vi "220125_xiang_calibration data analysis.vi"() -> ()   [LabVIEW 2020]
uses:
  OldDAQtask/CylinderCalibration/XYZE_power_spectra.ctl
  OldDAQtask/CylinderCalibration/single_power_spectrum.ctl
  OldDAQtask/CylinderCalibration/XYZ scan data.ctl
  OldDAQtask/CylinderCalibration/fast winding result.ctl
  <vilib>/Analysis/baseanly.llb/Mean (DBL).vi
  <vilib>/Utility/file.llb/Write Delimited Spreadsheet (DBL).vi
  OldDAQtask/HeightFinder/HeightFinder.lvlib
  <vilib>/Analysis/NI_AALBase.lvlib
  OldDAQtask/CylinderCalibration/CylinderCalibration.lvlib
  <vilib>/Analysis/NI_AALPro.lvlib
panel:
  out "ellipticity fitting 4":cluster{dbl[], dbl[]}[](graph)
  out "ellipticity fitting 3":cluster{dbl[], dbl[]}[](graph)
  out "ellipticity fitting 2":cluster{dbl[], dbl[]}[](graph)
  out "ellipticity fitting":cluster{dbl[], dbl[]}[](graph)
  out "error out":errorcluster
  out "pb1":dbl(slide)=1.0 scale=0.0..1.0
  in  "kT_pNnm":dbl=4.09
  in  "stop":bool
  in  "cylinder list":i32[](listbox)
  in  "root path":path=path "Y:/Setup4/xg237/220124_xg237_calibration Q30"
  in  "Tab Control":T1(tab)
  out "result":T2
  out "Height finder data":cluster{dbl[], "Best Polynomial Fit":dbl[]}[](graph)
  out "original calibration file":string="[Trap and cylinder calibration]\nKz, pN/nm/W=0.349554\nKx, pN/nm/W=0.376339\nKy, pN/nm/W=0.248999\nSz, 1/nm=0.000578\nSx, 1/nm=0.000761\nSy, 1/nm=0.000667\nKang, pNnm/rad/W=17149.300335\nMax ellipticity, 1=0.032157\nFocal shift=0.790000\nZsignalHeightDependence, 1/nm=0\n[Piezo AO calibration and settings]\nVx/Px(V/nm)=0.000667\nVy/Py(V/nm)=0.000667\nVz/Pz(V/nm)=0.002000\nMax Px (nm)=30000.000000\nMax Py (nm)=30000.000000\nMax Pz (nm)=10000.000000\nMin Px (nm)=0.000000\nMin Py (nm)=0.000000\nMin Pz (nm)=0.000000\nVx0 (V)=-10.000000\nVy0 (V)=-10.000000\nVz0 (V)=-10.000000\nAI2p=1.101000E+4\\095.746000E+3\\093.323000E+0\\0D\\0A1.016000E+4\\095.766000E+3\\093.739000E+0\\0D\\0A6.154000E+3\\095.319000E+3\\091.621000E+1\\0D\\0A\n[matrix Mp2s (3X3)]\na11=1.000000\na12=0.000000\na13=0.000000\na21=0.000000\na22=1.000000\na23=0.000000\na31=0.000000\na32=0.000000\na33=1.000000\n[DAQ settings]\nAIBufferSize=100000\nDAQ ScanRate=10000\nPoints to average=20\nSamping rate=500\n[PS detector signal to laser power (W) conversion matrix (2X2)]\na11=0.0152532\na12=-0.00000458129\na21=-0.0000113255\na22=0.0139626\n[Z bead vs Z signal polynomial coefficients (nm)]\na0=0.000000\na1=1773.000000\na2=0.000000\na3=0.000000\na4=0.000000\na5=0.000000\n[Z bead look up table]\n(Z signal, Z bead)=-1.000000E+2\\09-4.925198E+2\\0D\\0A-2.068564E-1\\09-4.740681E+2\\0D\\0A-2.031962E-1\\09-4.583933E+2\\0D\\0A-1.995359E-1\\09-4.445056E+2\\0D\\0A-1.958757E-1\\09-4.317229E+2\\0D\\0A-1.922155E-1\\09-4.195962E+2\\0D\\0A-1.885553E-1\\09-4.078497E+2\\0D\\0A-1.848951E-1\\09-3.963318E+2\\0D\\0A-1.812349E-1\\09-3.849767E+2\\0D\\0A-1.775747E-1\\09-3.737744E+2\\0D\\0A-1.739145E-1\\09-3.627475E+2\\0D\\0A-1.702543E-1\\09-3.519346E+2\\0D\\0A-1.665941E-1\\09-3.413777E+2\\0D\\0A-1.629339E-1\\09-3.311145E+2\\0D\\0A-1.592737E-1\\09-3.211728E+2\\0D\\0A-1.556135E-1\\09-3.115682E+2\\0D\\0A-1.519532E-1\\09-3.023034E+2\\0D\\0A-1.482930E-1\\09-2.933685E+2\\0D\\0A-1.446328E-1\\09-2.847427E+2\\0D\\0A-1.409726E-1\\09-2.763963E+2\\0D\\0A-1.373124E-1\\09-2.682934E+2\\0D\\0A-1.336522E-1\\09-2.603938E+2\\0D\\0A-1.299920E-1\\09-2.526561E+2\\0D\\0A-1.263318E-1\\09-2.450395E+2\\0D\\0A-1.226716E-1\\09-2.375059E+2\\0D\\0A-1.190114E-1\\09-2.300210E+2\\0D\\0A-1.153512E-1\\09-2.225562E+2\\0D\\0A-1.116910E-1\\09-2.150888E+2\\0D\\0A-1.080307E-1\\09-2.076026E+2\\0D\\0A-1.043705E-1\\09-2.000879E+2\\0D\\0A-1.007103E-1\\09-1.925414E+2\\0D\\0A-9.705012E-2\\09-1.849654E+2\\0D\\0A-9.338991E-2\\09-1.773671E+2\\0D\\0A-8.972970E-2\\09-1.697580E+2\\0D\\0A-8.606949E-2\\09-1.621523E+2\\0D\\0A-8.240929E-2\\09-1.545665E+2\\0D\\0A-7.874908E-2\\09-1.470176E+2\\0D\\0A-7.508887E-2\\09-1.395227E+2\\0D\\0A-7.142866E-2\\09-1.320976E+2\\0D\\0A-6.776845E-2\\09-1.247560E+2\\0D\\0A-6.410824E-2\\09-1.175090E+2\\0D\\0A-6.044804E-2\\09-1.103642E+2\\0D\\0A-5.678783E-2\\09-1.033255E+2\\0D\\0A-5.312762E-2\\09-9.639297E+1\\0D\\0A-4.946741E-2\\09-8.956269E+1\\0D\\0A-4.580720E-2\\09-8.282687E+1\\0D\\0A-4.214700E-2\\09-7.617425E+1\\0D\\0A-3.848679E-2\\09-6.959053E+1\\0D\\0A-3.482658E-2\\09-6.305893E+1\\0D\\0A-3.116637E-2\\09-5.656087E+1\\0D\\0A-2.750616E-2\\09-5.007675E+1\\0D\\0A-2.384595E-2\\09-4.358670E+1\\0D\\0A-2.018575E-2\\09-3.707141E+1\\0D\\0A-1.652554E-2\\09-3.051286E+1\\0D\\0A-1.286533E-2\\09-2.389508E+1\\0D\\0A-9.205121E-3\\09-1.720474E+1\\0D\\0A-5.544913E-3\\09-1.043171E+1\\0D\\0A-1.884705E-3\\09-3.569408E+0\\0D\\0A1.775503E-3\\093.384973E+0\\0D\\0A5.435712E-3\\091.043038E+1\\0D\\0A9.095920E-3\\091.756204E+1\\0D\\0A1.275613E-2\\092.477176E+1\\0D\\0A1.641634E-2\\093.204839E+1\\0D\\0A2.007654E-2\\093.937846E+1\\0D\\0A2.373675E-2\\094.674700E+1\\0D\\0A2.739696E-2\\095.413840E+1\\0D\\0A3.105717E-2\\096.153747E+1\\0D\\0A3.471738E-2\\096.893042E+1\\0D\\0A3.837759E-2\\097.630600E+1\\0D\\0A4.203779E-2\\098.365648E+1\\0D\\0A4.569800E-2\\099.097859E+1\\0D\\0A4.935821E-2\\099.827434E+1\\0D\\0A5.301842E-2\\091.055516E+2\\0D\\0A5.667863E-2\\091.128245E+2\\0D\\0A6.033884E-2\\091.201134E+2\\0D\\0A6.399904E-2\\091.274448E+2\\0D\\0A6.765925E-2\\091.348504E+2\\0D\\0A7.131946E-2\\091.423665E+2\\0D\\0A7.497967E-2\\091.500322E+2\\0D\\0A7.863988E-2\\091.578880E+2\\0D\\0A8.230008E-2\\091.659733E+2\\0D\\0A8.596029E-2\\091.743245E+2\\0D\\0A8.962050E-2\\091.829723E+2\\0D\\0A9.328071E-2\\091.919395E+2\\0D\\0A9.694092E-2\\092.012384E+2\\0D\\0A1.006011E-1\\092.108698E+2\\0D\\0A1.042613E-1\\092.208213E+2\\0D\\0A1.079215E-1\\092.310681E+2\\0D\\0A1.115818E-1\\092.415750E+2\\0D\\0A1.152420E-1\\092.523003E+2\\0D\\0A1.189022E-1\\092.632031E+2\\0D\\0A1.225624E-1\\092.742540E+2\\0D\\0A1.262226E-1\\092.854502E+2\\0D\\0A1.298828E-1\\092.968364E+2\\0D\\0A1.335430E-1\\093.085323E+2\\0D\\0A1.372032E-1\\093.207678E+2\\0D\\0A1.408634E-1\\093.339281E+2\\0D\\0A1.445236E-1\\093.486096E+2\\0D\\0A1.481838E-1\\093.656889E+2\\0D\\0A1.000000E+2\\093.864067E+2\\0D\\0A\n[Comment from Q30 Calibration] 10 mM Tris-HCl, pH = 8; 40 mM MgCl2; 50 mM NaCl; 0.2 mg/mL beta-casein\n1/14/2021 11:33 AM"
  out "Updated calibration file":string
  out "Updated calibration file location":path
  out "SD of force sensitivity, pN/W":dbl=12.607172653733816
  out "SEM of force sensitivity, pN/W":dbl=3.151793163433454
  out "mean force sensitivity, pN/W":dbl=492.26794237481425
  out "SD of torque sensitivity, pNnm/W":dbl=244140.75454887396
  out "SEM of torque sensitivity, pNnm/W":dbl=61035.18863721849
  out "mean torque sensitivity, pNnm/W":dbl=308105.85527126427
  out "SD of z stiffness, pN/nm/W":dbl=0.006440898726546468
  out "SD of z sensitivity, 1/nm":dbl=5.569909992065383e-06
  out "SD of angular stifness, pNnm/rad/W":dbl=320.0752807876521
  out "SD of angular sensitivity, 1/rad":dbl=0.00035066082703313163
  out "z force sensitivity":T3(graph)={"final result"=[1.0, 2.0, 3.0, 4.0, 6.0, 7.0], "final result"=[498.4071904780335, 474.8213008025603, 504.1808261472068, 495.5040400134854, 478.2463154671384, 502.4479813404608]}
  out "Torque sensitivity":T3(graph)={"final result"=[1.0, 2.0, 3.0, 4.0, 6.0, 7.0], "final result"=[73.67021354183011, -8913.301705379306, 498179.1915137824, 417955.8385778271, 442478.0259262357, 498861.70710157783]}
  out "SEM of z stiffness, pN/nm/W":dbl=0.001610224681636617
  out "mean z stiffness, pN/nm/W":dbl=0.16169724642273595
  out "SEM of z sensitivity, 1/nm":dbl=1.3924774980163457e-06
  out "mean z sensitivity, 1/nm":dbl=0.00032838353115096313
  out "SEM of angular stifness, pNnm/rad/W":dbl=80.01882019691303
  out "mean angular stiffness, pNnm/rad/W":dbl=375.5197105345397
  out "SEM of angular sensitivity, 1/rad":dbl=8.766520675828291e-05
  out "mean angular sensitivity, 1/rad":dbl=0.0013622152574613259
  out "final result":dbl[][](array[numeric])=[[1.0, 2.0, 3.0, 4.0, 6.0, 7.0], [nan, nan, nan, nan, nan, nan], [0.13279234841776086, -13.36709953944761, 674.8537139952265, 372.11897404124767, 711.6919827860539, 507.68789957574], [0.0018025242772285583, 0.001499679914501309, 0.0013546405098627172, 0.0008903308428647679, 0.0016084233364951283, 0.001017692663815475], [73.67021354183011, -8913.301705379306, 498179.1915137824, 417955.8385778271, 442478.0259262357, 498861.70710157783], [0.16579227343626485, 0.1513303954658166, 0.16883942461520451, 0.16284381884534085, 0.15689235695361436, 0.16448520922017446], [0.00033264422464942726, 0.00031871020784036524, 0.0003348787098974448, 0.00032864276715263306, 0.0003280576386675683, 0.00032736763869834043], [498.4071904780335, 474.8213008025603, 504.1808261472068, 495.5040400134854, 478.2463154671384, 502.4479813404608], [0.6695465077566299, 0.9654608095555708, 1.1766726492381052, 1.2199767576089258, 1.1806760501666687, 0.7481024842794938], [0.0006195077361526612, 0.0007552886971877524, 0.0008161495017131666, 0.0008342978728837841, 0.0008284250298047227, 0.0006508474644543304], [1080.771826861639, 1278.267254826366, 1441.7366509054655, 1462.279597324187, 1425.205670626561, 1149.428284101409], [0.7539490293969152, 0.9600841428867122, 1.1413404013712398, 1.013487614262731, 1.027256013548298, 0.8640080844160597], [0.0005940302228699274, 0.0006707172355041432, 0.0007217134695992056, 0.0007028215814044456, 0.000725406642994016, 0.0006430202724935601], [1269.2098825449907, 1431.4290614062822, 1581.4314813953365, 1442.0268828932126, 1416.1105684233055, 1343.6716093965963], [0.19148344824695612, 0.21192606642906414, 0.19576149623991493, 0.19479979524743082, 0.19336718080202564, 0.19576422973039367], [0.12166886063179862, 0.12359792221219097, 0.12170898606033095, 0.12101974277514069, 0.11972394587250185, 0.12216359051715364]]
  out "z sensitivity":T3(graph)={"final result"=[1.0, 2.0, 3.0, 4.0, 6.0, 7.0], "final result"=[0.00033264422464942726, 0.00031871020784036524, 0.0003348787098974448, 0.00032864276715263306, 0.0003280576386675683, 0.00032736763869834043]}
  out "Angular sensitivity":T3(graph)={"final result"=[1.0, 2.0, 3.0, 4.0, 6.0, 7.0], "final result"=[0.0018025242772285583, 0.001499679914501309, 0.0013546405098627172, 0.0008903308428647679, 0.0016084233364951283, 0.001017692663815475]}
  out "max z force, pN/W":dbl=97.02091670635467
  out "SEM of max z force, pN/W":dbl=0.7160625967795665
  out "SD of max z force, pN/W":dbl=2.864250387118266
  out "Maximum torque":T3(graph)={"final result"=[1.0, 2.0, 3.0, 4.0, 6.0, 7.0], "final result"=[0.06639617420888043, -6.683549769723805, 337.42685699761324, 186.05948702062383, 355.84599139302696, 253.84394978787]}
  out "Maximum z force":T3(graph)={"final result"=[1.0, 2.0, 3.0, 4.0, 6.0, 7.0], "final result"=[95.43672746381132, 100.62701053581804, 98.69919290205362, 96.52408553890173, 92.47714175083674, 98.36134204670653]}
  out "Angular stiffness":T3(graph)={"final result"=[1.0, 2.0, 3.0, 4.0, 6.0, 7.0], "final result"=[0.13279234841776086, -13.36709953944761, 674.8537139952265, 372.11897404124767, 711.6919827860539, 507.68789957574]}
  out "z stiffness":T3(graph)={"final result"=[1.0, 2.0, 3.0, 4.0, 6.0, 7.0], "final result"=[0.16579227343626485, 0.1513303954658166, 0.16883942461520451, 0.16284381884534085, 0.15689235695361436, 0.16448520922017446]}
  out "CV of max z force":dbl=0.029521988498493166
  out "CV of angular sensitivity":dbl=0.2574195415243226
  out "CV of angular stifness":dbl=0.8523528108072828
  out "CV of z sensitivity":dbl=0.016961599665315758
  out "CV of z stiffness":dbl=0.03983307612862866
  out "CV of torque sensitivity":dbl=0.7923924533466792
  out "CV of force sensitivity":dbl=0.02561038728809742
  out "mean":dbl[](array[numeric])=[3.8333333333333335, nan, 375.5197105345397, 0.0013622152574613259, 308105.85527126427, 0.16169724642273595, 0.00032838353115096313, 492.26794237481425, 0.9934058764342324, 0.0007507527170327362, 1306.2815474409379, 0.960020880980326, 0.0006762849041442163, 1413.9799143432874, 0.1971837027826309, 0.12164717467818613]
  out "sd":dbl[](array[numeric])=[2.3166067138525404, nan, 320.0752807876521, 0.00035066082703313163, 244140.75454887396, 0.006440898726546468, 5.569909992065383e-06, 12.607172653733816, 0.2390944431916935, 9.435719400130207e-05, 163.137245645585, 0.13560242786564763, 5.115518013146681e-05, 104.91643534205578, 0.007404277385621852, 0.0012781918494249795]
  out "x stiffness":T3(graph)={"final result"=[1.0, 2.0, 3.0, 4.0, 6.0, 7.0], "final result"=[0.6695465077566299, 0.9654608095555708, 1.1766726492381052, 1.2199767576089258, 1.1806760501666687, 0.7481024842794938]}
  out "Maximum x force":T3(graph)={"final result"=[1.0, 2.0, 3.0, 4.0, 6.0, 7.0], "final result"=[60.64063499615816, 58.68692620128618, 61.36333714143654, 59.96577146647502, 57.25753598671112, 61.38084944864651]}
  out "x sensitivity":T3(graph)={"final result"=[1.0, 2.0, 3.0, 4.0, 6.0, 7.0], "final result"=[0.0006195077361526612, 0.0007552886971877524, 0.0008161495017131666, 0.0008342978728837841, 0.0008284250298047227, 0.0006508474644543304]}
  out "x force sensitivity":T3(graph)={"final result"=[1.0, 2.0, 3.0, 4.0, 6.0, 7.0], "final result"=[1080.771826861639, 1278.267254826366, 1441.7366509054655, 1462.279597324187, 1425.205670626561, 1149.428284101409]}
  out "max x force, pN/W":dbl=59.882509206785585
  out "SD of max x force, pN/W":dbl=1.6333686233039957
  out "SEM of max x force, pN/W":dbl=0.4083421558259989
  out "CV of max x force":dbl=0.027276222137981327
  out "mean x stiffness, pN/nm/W":dbl=0.9934058764342324
  out "SEM of x stiffness, pN/nm/W":dbl=0.05977361079792338
  out "SD of x stiffness, pN/nm/W":dbl=0.2390944431916935
  out "CV of x stiffness":dbl=0.24068152692020295
  out "mean z sensitivity, 1/nm 2":dbl=0.0007507527170327362
  out "SEM of z sensitivity, 1/nm 2":dbl=2.358929850032552e-05
  out "SD of z sensitivity, 1/nm 2":dbl=9.435719400130207e-05
  out "CV of z sensitivity 2":dbl=0.1256834532337599
  out "Comment":string
  out "Name":string
  out "data":T4(array[cluster])
  out "Array":dbl[][](array[numeric])
  in  "psd fitting ranges":T5(array[cluster])=[{"Angle High frequency cutoff %"=95.0, "z High frequency cutoff %"=70.0, "x High frequency cutoff %"=50.0, "y High frequency cutoff %"=50.0}, {"Angle High frequency cutoff %"=95.0, "z High frequency cutoff %"=70.0, "x High frequency cutoff %"=50.0, "y High frequency cutoff %"=50.0}, {"Angle High frequency cutoff %"=90.0, "z High frequency cutoff %"=70.0, "x High frequency cutoff %"=50.0, "y High frequency cutoff %"=50.0}, {"Angle High frequency cutoff %"=80.0, "z High frequency cutoff %"=70.0, "x High frequency cutoff %"=50.0, "y High frequency cutoff %"=50.0}]
  in  "import?":bool
  in  "fast winding results":T6[](array[typedef]) {"Laser power before obj[W]" format="%.4f"; "relative fluctuation (fluctuation/mean)" format="%#_6e"; "mean e amplitude" format="%#_6e"}
  in  "stifness results":T7[][](array[typedef]) {"result of y signal"."var" format="%.3e"; "result of y signal"."sigma^2" format="%.3e"; "result of x signal"."var" format="%.3e"; "result of x signal"."sigma^2" format="%.3e"; "result of z signal"."var" format="%.3e"; "result of z signal"."sigma^2" format="%.3e"; "result of ellipticity"."var" format="%.3e"; "result of ellipticity"."sigma^2" format="%.3e"; "general info"."Time/Date" format="%<%.3X, %x>T"}
  in  "XYZ scan result":T9 {"y_signal vs trap height slope around eq position, 1/nm" format="%#.6g"; "x_signal vs trap height slope around eq position, 1/nm" format="%#.6g"; "Zsig baseline" format="%#.6g"; "Xsig baseline" format="%#.6g"; "Ysig baseline" format="%#.6g"; "z_signal vs trap height slope around eq position, 1/nm" format="%#.6g"}
  out "only use slopes":dbl[][](array[numeric]) format="%_3e"
  out "intercepts that will be ignored":dbl[][](array[numeric]) format="%_3e"
  out "distance between trap center and z DoG center":dbl
  # "Rows:\n\n0: Cylinder No.\n1: \n2: K_theta\n3: S_theta\n4: K_e\n5: K_z\n6: S_z\n7: K_zsig\n8: K_x\n9: S_x\n10: K_xsig\n11: K_y\n12: S_y\n13: K_ysig\n14: Max z signal\n15: Max x signal"
  # "column name:\n\n0: Cylinder No.\n1: Good? (=1)\n2: K_theta\n3: S_theta\n4: K_e\n5: K_z\n6: S_z\n7: K_zsig\n8: K_x\n9: S_x\n10: K_xsig\n11: K_y\n12: S_y\n13: K_ysig\n14: Max z signal\n15: Max x signal"
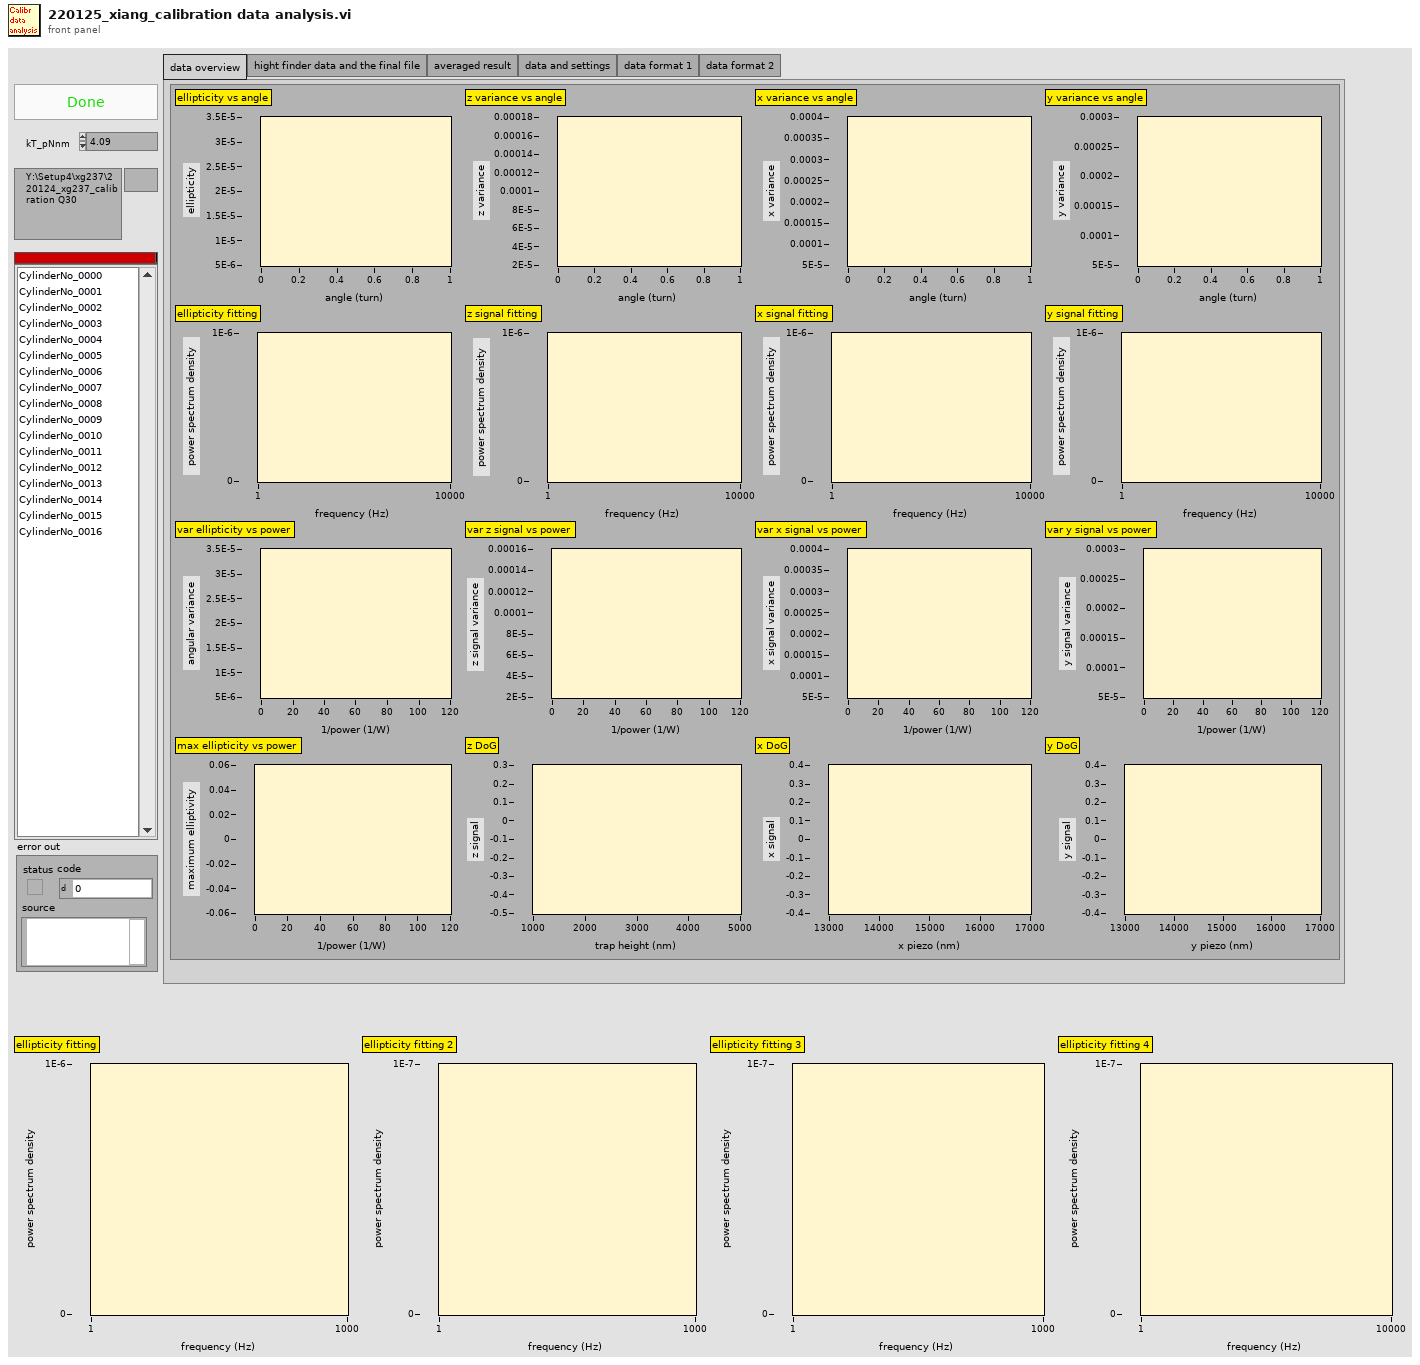
[diagram p1: front panel]
types:
  T1 = enum32{"data overview", "hight finder data and the final file", "averaged result", "data and settings", "data format 1", "data format 2"}
  T2 = cluster{"max ellipticity vs power":cluster{dbl[], dbl[]}[], "z DoG":cluster{dbl[], dbl[]}[], "x DoG":cluster{dbl[], dbl[]}[], "y DoG":cluster{dbl[], dbl[]}[], "ellipticity vs angle":cluster{dbl[], dbl[]}[], "z variance vs angle":cluster{dbl[], dbl[]}[], "x variance vs angle":cluster{dbl[], dbl[]}[], "y variance vs angle":cluster{dbl[], dbl[]}[], "var ellipticity vs power":cluster{dbl[], dbl[]}[], "var z signal vs power":cluster{dbl[], dbl[]}[], "var x signal vs power":cluster{dbl[], dbl[]}[], "var y signal vs power":cluster{dbl[], dbl[]}[], "ellipticity fitting":cluster{dbl[], dbl[]}[], "z signal fitting":cluster{dbl[], dbl[]}[], "x signal fitting":cluster{dbl[], dbl[]}[], "y signal fitting":cluster{dbl[], dbl[]}[]}
  T3 = cluster{"final result":dbl[], "final result":dbl[]}
  T4 = cluster{i32, cluster{"Y":dbl[], "Y":dbl[]}, cluster{dbl[], dbl[]}, cluster{dbl[], "Best Polynomial Fit":dbl[]}, cluster{dbl[], "Best Polynomial Fit":dbl[]}, cluster{dbl[], "Best Polynomial Fit":dbl[]}, dbl[], cluster{dbl[], dbl[]}[], cluster{dbl[], dbl[]}[], cluster{dbl[], dbl[]}[], cluster{dbl[], dbl[]}[], cluster{dbl, dbl}, cluster{dbl[], dbl[]}, cluster{dbl[], dbl[]}, cluster{dbl[], dbl[]}, cluster{dbl[], dbl[]}, cluster{dbl[], "best nonlinear fit":dbl[]}[], cluster{dbl[], "best nonlinear fit":dbl[]}[], cluster{dbl[], "best nonlinear fit":dbl[]}[], cluster{dbl[], "best nonlinear fit":dbl[]}[], "var of linear fittings":dbl[][]}[]
  T5 = cluster{"Angle High frequency cutoff %":dbl, "z High frequency cutoff %":dbl, "x High frequency cutoff %":dbl, "y High frequency cutoff %":dbl}[]
  T6 = typedef "CylinderCalibration.lvlib/fast winding result.ctl" = cluster{"fast pol (current file)":dbl[], "fit fast pol fitting result":cluster{dbl[], "best nonlinear fit":dbl[]}[], "fit result: amplitude":dbl[], "mean e amplitude":dbl, "relative fluctuation (fluctuation/mean)":dbl, "Laser power before obj[W]":dbl}
  T7 = typedef "CylinderCalibration.lvlib/XYZE_power_spectra.ctl" = cluster{"general info":cluster{"Time/Date ":timestamp, "Laser power before obj[W]":dbl, "Cylinder height  [nm]":dbl, "Polarization angle (turn)":dbl}, "result of ellipticity":T8, "result of z signal":T8, "result of x signal":T8, "result of y signal":T8}
  T8 = typedef "CylinderCalibration.lvlib/single_power_spectrum.ctl" = cluster{"raw signal (linear drift removed)":dbl[], "signal distribution":cluster{"X Values":dbl[], "Best Gaussian Fit":dbl[]}[], "power":cluster{dbl[], "best nonlinear fit":dbl[]}[], "A and fc":dbl[], "cutoff %":dbl, "dt [s] ":dbl, "sigma^2":dbl, "var ":dbl}
  T9 = typedef "CylinderCalibration.lvlib/XYZ scan data.ctl" = cluster{"height finder result":cluster{"Y":dbl[], "Y":dbl[]}[], "Instrument Calibr.XYZsignal baseline.Zsignal0":dbl, "Z signal vs trap height, fitting":cluster{dbl[], "Best Polynomial Fit":dbl[]}[], "z_signal vs trap height slope around eq position, 1/nm":dbl, "Z signal Truncated data with redrawn polynomial":cluster{dbl[], "Best Polynomial Fit":dbl[]}[], "Z signal Residues":cluster{dbl[], dbl[]}, "Z center positon":dbl, "Zsig baseline":dbl, "X signal Truncated data with redrawn polynomial":cluster{dbl[], "Best Polynomial Fit":dbl[]}[], "X signal Residues":cluster{dbl[], dbl[]}, "X center positon":dbl, "Xsig baseline":dbl, "Y signal Truncated data with redrawn polynomial":cluster{dbl[], "Best Polynomial Fit":dbl[]}[], "Y signal Residues":cluster{dbl[], dbl[]}, "Y center positon":dbl, "Ysig baseline":dbl, "x_signal vs trap height slope around eq position, 1/nm":dbl, "y_signal vs trap height slope around eq position, 1/nm":dbl}
  T10 = enum16{"deny read/write", "deny write-only", "deny none"}
  T11 = typedef "lveventtype.ctl" = enum32{"Null", "Timeout", "Annotation Menu Selection", "Annotation Menu Selection?", "App Instance Close", "App Instance Close?", "Autoscale Range Change", "Bookmark Info Change", "Cell Edit", "Cell Edit?", "Cursor Grab", "Cursor Grab?", "Cursor Menu Selection", "Cursor Menu Selection?", "Cursor Move", "Cursor Release", "Data Change", "Direction Change", "Display State Change", "Drag Ended", "Drag Enter", "Drag Leave", "Drag Over", "Drag Source Update", "Drag Starting", "Drag Starting?", "Drop", "Exec State Change", "Key Down", "Key Down?", "Key Repeat", "Key Repeat?", "Key Up", "Listbox Double Click", "Menu Activation?", "Menu Selection (App)", "Menu Selection? (App)", "Menu Selection (User)", "Mouse Down", "Mouse Down?", "Mouse Enter", "Mouse Leave", "Mouse Move", "Mouse Up", "Mouse Wheel", "NI Security User Change (App)", "Pane Size", "Panel Close", "Panel Close?", "Panel Resize", "Plot Attribute Change", "Scale Range Change", "Shortcut Menu Activation?", "Shortcut Menu Selection (App)", "Shortcut Menu Selection? (App)", "Shortcut Menu Selection (User)", "Tree Double Click", "Tree Drag", "Tree Drag?", "Tree Drop", "Tree Drop?", "Tree Item Close", "Tree Item Close?", "Tree Item Open", "Tree Item Open?", "User Event", "Value Change"}
  T12 = cluster{"A":dbl, "f0":dbl, "pi A^2/f0":dbl, "k domain":cluster{dbl[], "best nonlinear fit":dbl[]}[]}
  T13 = cluster{i32, cluster{"Y":dbl[], "Y":dbl[]}, cluster{dbl[], dbl[]}, cluster{dbl[], "Best Polynomial Fit":dbl[]}, cluster{dbl[], "Best Polynomial Fit":dbl[]}, cluster{dbl[], "Best Polynomial Fit":dbl[]}, dbl[], cluster{dbl[], dbl[]}[], cluster{dbl[], dbl[]}[], cluster{dbl[], dbl[]}[], cluster{dbl[], dbl[]}[], cluster{dbl, dbl}, cluster{dbl[], dbl[]}, cluster{dbl[], dbl[]}, cluster{dbl[], dbl[]}, cluster{dbl[], dbl[]}, cluster{dbl[], "best nonlinear fit":dbl[]}[], cluster{dbl[], "best nonlinear fit":dbl[]}[], cluster{dbl[], "best nonlinear fit":dbl[]}[], cluster{dbl[], "best nonlinear fit":dbl[]}[], dbl[][]}
  T14 = cluster{i32, cluster{"Y":dbl[], "Y":dbl[]}, cluster{dbl[], dbl[]}, cluster{dbl[], "Best Polynomial Fit":dbl[]}, cluster{dbl[], "Best Polynomial Fit":dbl[]}, cluster{dbl[], "Best Polynomial Fit":dbl[]}, dbl[], cluster{dbl[], dbl[]}[], cluster{dbl[], dbl[]}[], cluster{dbl[], dbl[]}[], cluster{dbl[], dbl[]}[], cluster{dbl, dbl}, cluster{dbl[], dbl[]}, cluster{dbl[], dbl[]}, cluster{dbl[], dbl[]}, cluster{dbl[], dbl[]}, cluster{dbl[], "best nonlinear fit":dbl[]}[], cluster{dbl[], "best nonlinear fit":dbl[]}[], cluster{dbl[], "best nonlinear fit":dbl[]}[], cluster{dbl[], "best nonlinear fit":dbl[]}[], "var of linear fittings":dbl[][]}
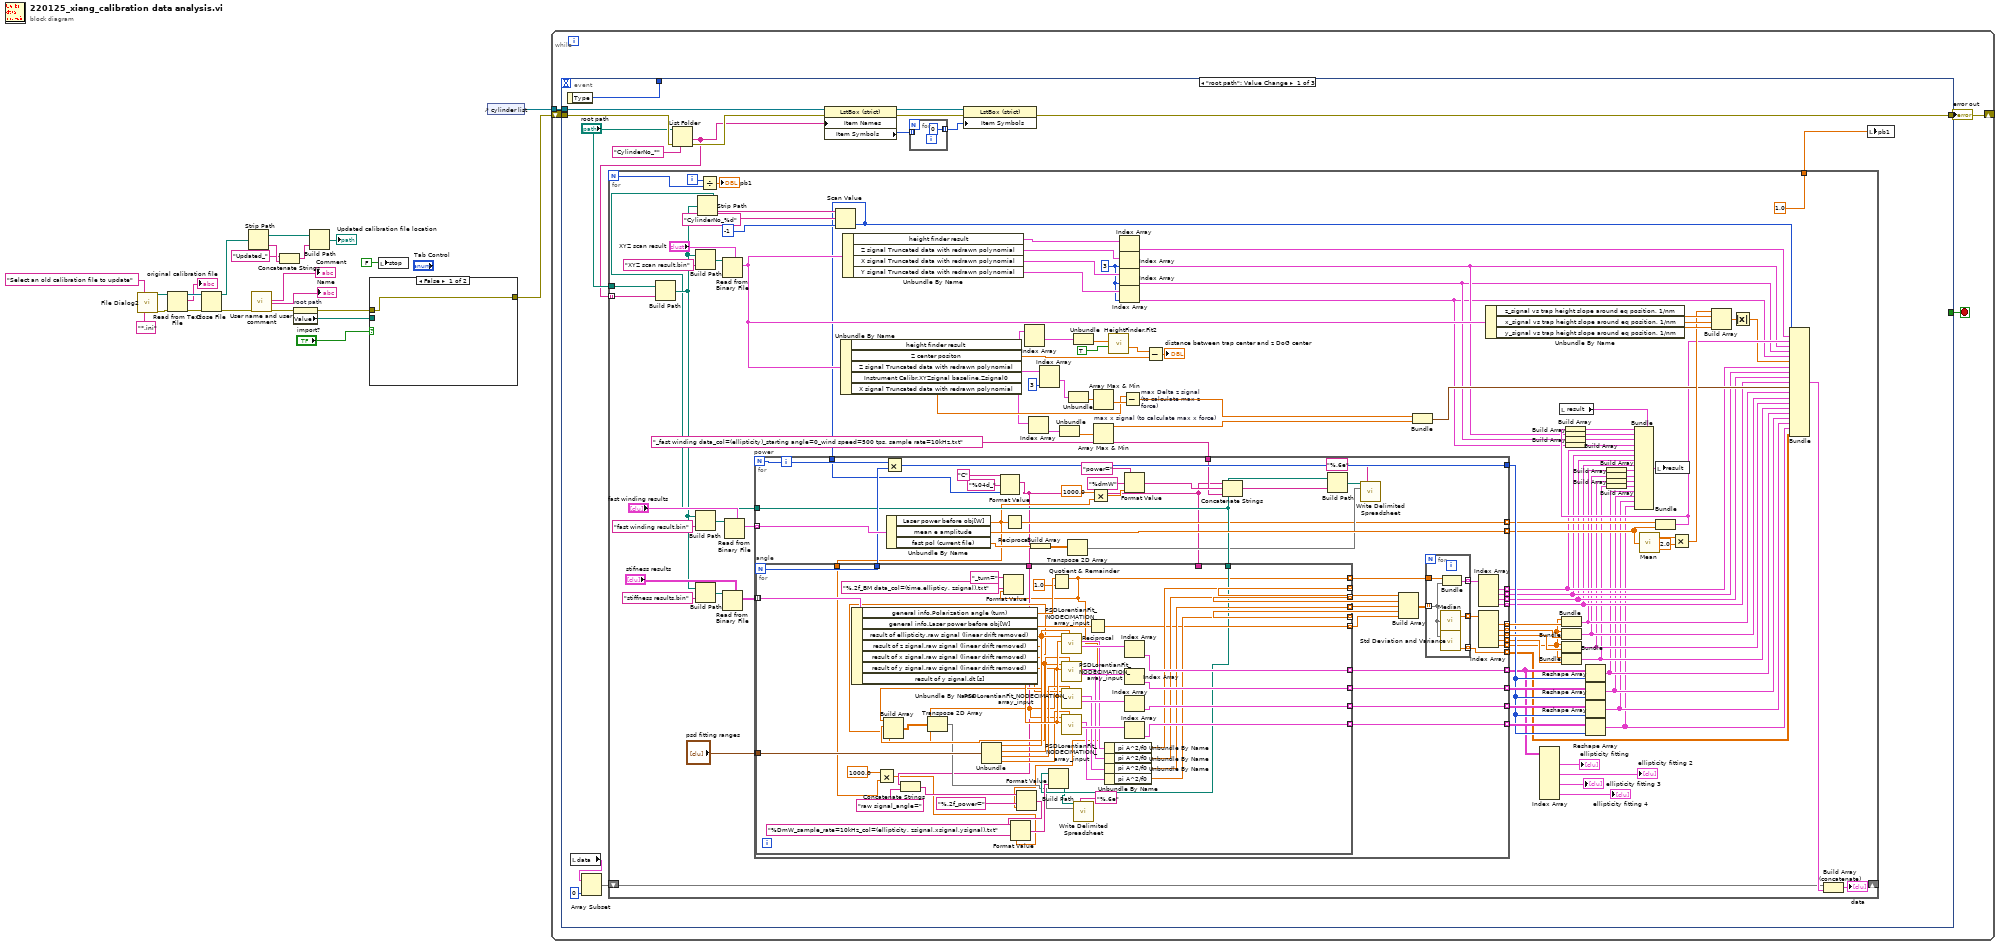
[diagram p0: block diagram]
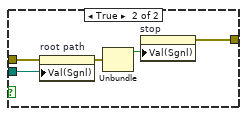
[diagram p2: hidden frame]
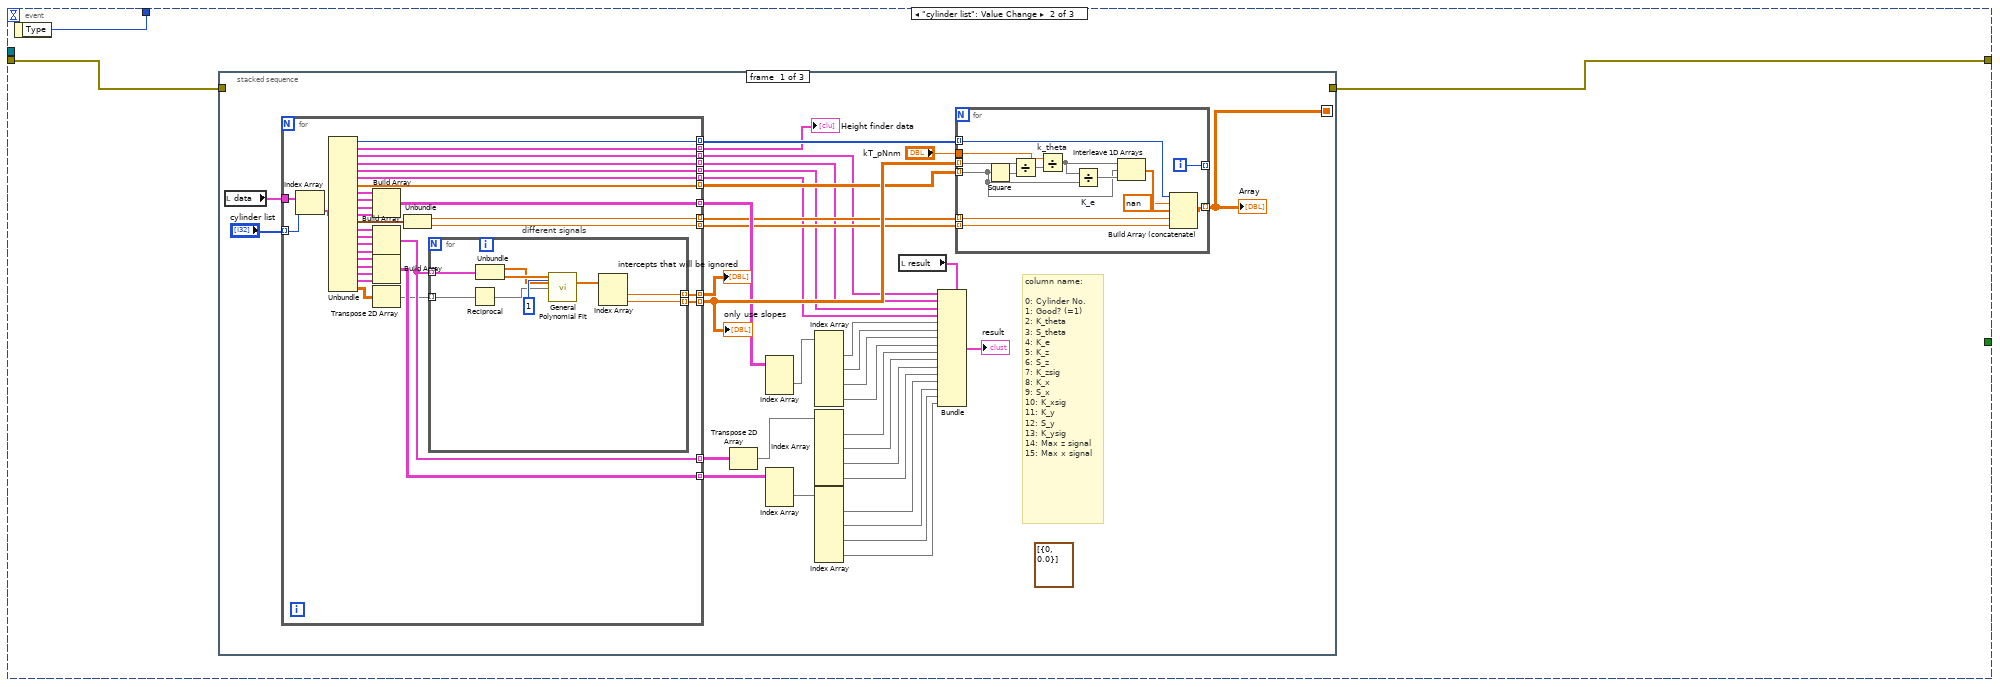
[diagram p3: hidden frame]
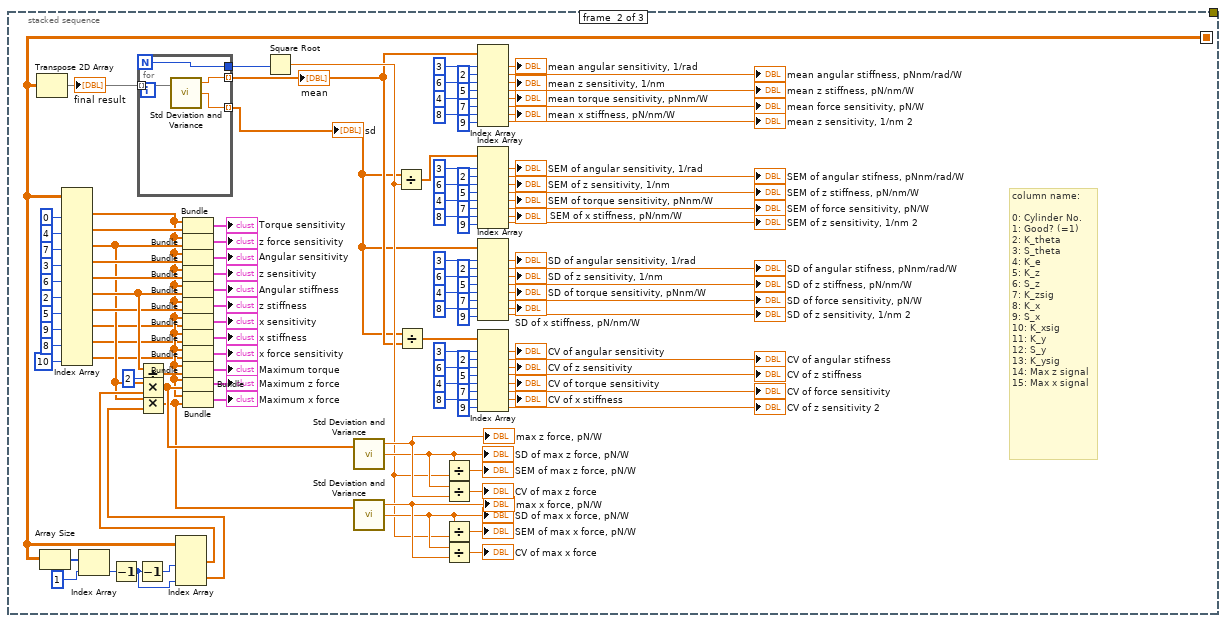
[diagram p4: hidden frame]
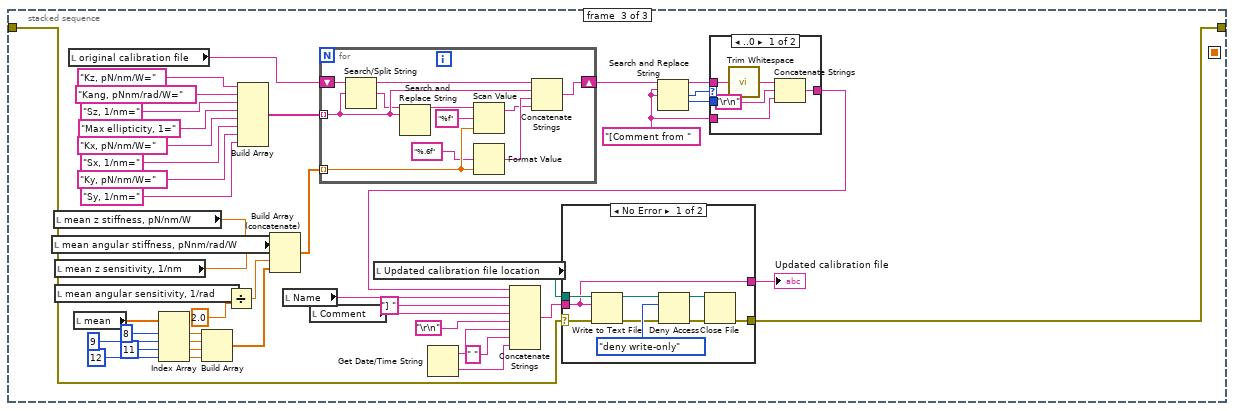
[diagram p5: hidden frame]
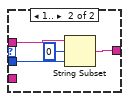
[diagram p6: hidden frame]
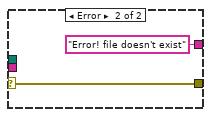
[diagram p7: hidden frame]
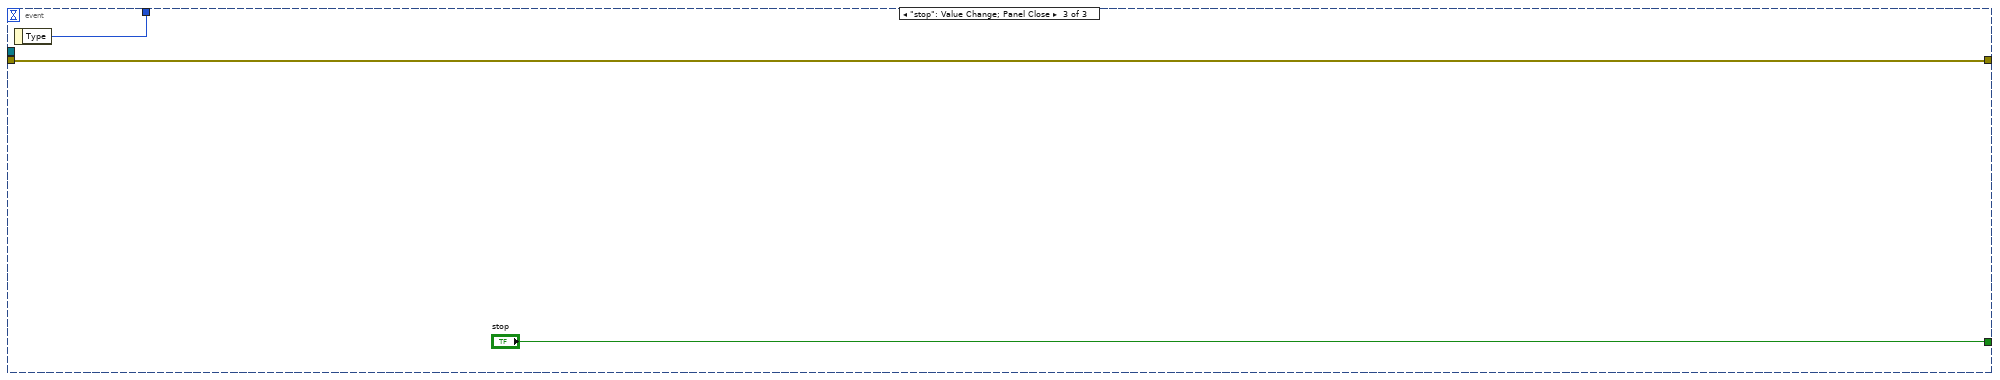
[diagram p8: hidden frame]
diagram:
  n1 = call "File Dialog2"("prompt"="Select an old calibration file to update", "pattern (all files)"="*.ini") -> ("selected path"=w18:path, "error out"=w9:errorcluster)  [unwired: 10 in, 2 out]
  n2 = Read from Text File(file (use dialog)=w18, error in=w9) -> (refnum out=w20:refnum<file>, text=→"original calibration file":string, error out=w17:errorcluster)  [unwired: 2 in, 1 out]
  n3 = Close File(refnum=w20, error in=w17) -> (path=w8:path, error out=w4:errorcluster)
  n4 = Strip Path(path=w8) -> (stripped path=w11:path, name=w13:string)
  n5 = call "User name and user comment"("error in (no error)"=w4) -> ("Comment"=→"Comment":string, "Name"=→"Name":string, "error out"=w3:errorcluster)  [unwired: 15 in, 1 out]
  n6 = Concatenate Strings("Updated_" ("name"), w13) -> (w14:string)
  n7 = property on="root path" class="Path"(error in=w3) -> (error out=w23:errorcluster, "Value"=w22:path)  [unwired: 1 in, 1 out]
  n8 = Build Path(base path=w11, name or relative path=w14) -> (appended path=→"Updated calibration file location":path)
  n9 = case shown="False" "import?" {
    tunnel: w23 -> [w24 w29]
    tunnel: w22 -> [_ w28]
    tunnel: [w24 w25] -> w2
    frame False {
    }
    frame True {
      n10 = property on="root path" class="Path"(error in=w29, "Val(Sgnl)"=w28) -> (error out=w27:errorcluster)  [unwired: 1 in, 1 out]
      n11 = Unbundle(w27) -> ("status"=w26:bool)  [unwired: 2 out]
      n12 = property on="stop" class="Bool (strict)"("Val(Sgnl)"=w26) -> (error out=w25:errorcluster)  [unwired: 2 in, 1 out]
    }
  }
  n13 = local write "stop"(FALSE ("stop")) -> ()
  n14 = control-ref of="cylinder list"() -> (w5:refnum<vi>)
  n15 = while {
    shift-right: [w30] -> _
    shift-left: w2 -> [w33]
    tunnel: w5 -> [w31]
    stop <- w32 stop-if-true
    n16 = event shown="[0] \"root path\": Value Change" {
      selector: _ -> [_ _ _]
      dyn-events: _ -> [_ _ _]
      timeout: _ -> [_ _ _]
      tunnel: w31 -> [w44 _ _]
      tunnel: w33 -> [w43 w262 w557]
      tunnel: [_ _ "stop"] -> w32
      tunnel: [w40 w261 w557] -> w30
      tunnel: [w41 w260 w556] -> _
      event "root path": Value Change {
        n17 = event-data() -> ("Type"=w41:T11)  [unwired: 1 in]
        n18 = local read "data"() -> (w35:T4)
        n19 = Array Subset(array=w35, length=0) -> (w38:T4)  [unwired: 1 in]
        n20 = List Folder(path="root path", pattern="CylinderNo_*", error in=w43) -> (folder names=w36:string[], error out=w42:errorcluster)  [unwired: 1 in, 2 out]
        n21 = for {
          N -> [w127]
          shift-right: [w97] -> _
          shift-left: w38 -> [w96]
          tunnel: [1.0 ("pb1")] -> w39
          tunnel: w36 -> [w93] mode=indexing
          tunnel: "root path" -> [w94]
          i -> [w125]
          w126 = 3 ("index")
          n22 = Build Path(base path=w94, name or relative path=w93) -> (appended path=w92:path)
          n23 = Build Path(base path=w92, name or relative path="fast winding result.bin") -> (appended path=w153:path)
          n24 = Build Path(base path=w92, name or relative path="XYZ scan result.bin") -> (appended path=w152:path)
          n25 = Build Path(base path=w92, name or relative path="stiffness results.bin") -> (appended path=w154:path)
          n26 = Strip Path(path=w92) -> (stripped path=w52:path, name=w53:string)
          n27 = Divide(x=w125, y=w127) -> (x/y=→"pb1":dbl)
          n28 = Read from Binary File(5:"XYZ scan result", 11:w152) -> (2:w106:T9)  [unwired: 4 in, 3 out]
          n29 = Read from Binary File(5:"stifness results", 11:w154) -> (2:w147:T7[][])  [unwired: 4 in, 3 out]
          n30 = Read from Binary File(5:"fast winding results", 11:w153) -> (2:w146:T6[])  [unwired: 4 in, 3 out]
          n31 = Scan Value(string=w53, format string="CylinderNo_%d" ("pattern"), default (0 dbl)=-1) -> (value=w51:i32)  [unwired: 1 out]
          n32 = for "power" {
            N -> [w182]
            tunnel: w147 -> [w203] mode=indexing
            tunnel: w146 -> [w202] mode=indexing
            tunnel: [w193] -> w80 mode=indexing
            tunnel: [w192] -> w79 mode=indexing
            tunnel: [w191] -> w78 mode=indexing
            tunnel: [w190] -> w77 mode=indexing
            tunnel: [w188] -> w62 mode=indexing
            tunnel: [w187] -> w63 mode=indexing
            tunnel: [w186] -> w140 mode=indexing
            tunnel: [w185] -> w141 mode=indexing
            tunnel: [w184] -> w142 mode=indexing
            tunnel: [w181] -> w136
            tunnel: [w180] -> w61 mode=indexing
            tunnel: [w179] -> w139 mode=indexing
            tunnel: [w178] -> w138 mode=indexing
            tunnel: [w177] -> w137 mode=indexing
            tunnel: [w161] -> w129 mode=indexing
            tunnel: [w176] -> w124 mode=indexing
            tunnel: "psd fitting ranges" -> [w175] mode=indexing
            tunnel: [w174] -> w54 mode=indexing
            tunnel: w52 -> [w172]
            tunnel: w51 -> [w166]
            tunnel: "_fast winding data_col=(ellipticity)_starting angle=0_wind speed=500 tps, sample rate=10kHz.txt" ("string") -> [w159]
            n33 = Unbundle By Name(w202) -> ("Laser power before obj[W]"=w156:dbl, "mean e amplitude"=w176:dbl, "fast pol (current file)"=w169:dbl[])
            n34 = Format Value(string ("")="C", format string="%04d_", value (0)=w166) -> (output string=w155:string)
            n35 = for "angle" {
              N -> [w258]
              tunnel: w203 -> [w255] mode=indexing
              tunnel: [w236] -> w197 mode=indexing
              tunnel: [w235] -> w198 mode=indexing
              tunnel: [w234] -> w199 mode=indexing
              tunnel: [w233] -> w201 mode=indexing
              tunnel: [w232] -> w195 mode=indexing
              tunnel: [w209] -> w200 mode=indexing
              tunnel: [w246] -> w177 mode=indexing
              tunnel: [w247] -> w178 mode=indexing
              tunnel: [w248] -> w179 mode=indexing
              tunnel: [w249] -> w180 mode=indexing
              tunnel: [w258] -> w183
              tunnel: w175 -> [w237]
              tunnel: w172 -> [w219]
              tunnel: w155 -> [_]
              tunnel: w156 -> [w211]
              tunnel: w155 -> [w215]
              n36 = Unbundle By Name(w255) -> ("general info.Polarization angle (turn)"=w257:dbl, "general info.Laser power before obj[W]"=w229:dbl, "result of ellipticity.raw signal (linear drift removed)"=w228:dbl[], "result of z signal.raw signal (linear drift removed)"=w227:dbl[], "result of x signal.raw signal (linear drift removed)"=w226:dbl[], "result of y signal.raw signal (linear drift removed)"=w225:dbl[], "result of y signal.dt [s]"=w254:dbl)
              n37 = Multiply(x=1000.0, y=w211) -> (x*y=w210:dbl)
              n38 = Build Array(w228, w227, w226, w225) -> (w224:dbl[][])
              n39 = Concatenate Strings(w215, "raw signal_angle=" ("string (\"\")")) -> (w213:string)
              n40 = Transpose 2D Array(2D array=w224) -> (transposed array=w216:dbl[][])
              n41 = Unbundle(w237) -> ("Angle High frequency cutoff %"=w241:dbl, "z High frequency cutoff %"=w240:dbl, "x High frequency cutoff %"=w239:dbl, "y High frequency cutoff %"=w238:dbl)
              n42 = Quotient & Remainder(x=w257, y=1.0) -> (x-y*floor(x/y)=w209:dbl)  [unwired: 1 out]
              n43 = Format Value(string ("")="_turn=", format string="%.2f_BM data_col=(time,ellipticy, zsignal).txt", value (0)=w209) -> ()  [unwired: 1 out]
              n44 = Format Value(string ("")=w213, format string="%.2f_power=", value (0)=w209) -> (output string=w221:string)
              n45 = Format Value(string ("")=w221, format string="%DmW_sample_rate=10kHz_col=(ellipticity, zsignal,xsignal,ysignal).txt", value (0)=w210) -> (output string=w220:string)
              n46 = Build Path(base path=w219, name or relative path=w220) -> (appended path=w218:path)
              n47 = call "PSDLorentianFit_NODECIMATION_array_input.vi"("High frequency cutoff %"=w241, "dt [s]"=w254, "signal"=w228) -> ("k domain resampled"=w253:cluster{dbl[], "best nonlinear fit":dbl[]}[], "frequency domain info"=w245:T12)  [unwired: 5 in, 2 out]
              n48 = call "PSDLorentianFit_NODECIMATION_array_input.vi"("High frequency cutoff %"=w240, "dt [s]"=w254, "signal"=w227) -> ("k domain resampled"=w250:cluster{dbl[], "best nonlinear fit":dbl[]}[], "frequency domain info"=w244:T12)  [unwired: 5 in, 2 out]
              n49 = call "PSDLorentianFit_NODECIMATION_array_input.vi"("High frequency cutoff %"=w239, "dt [s]"=w254, "signal"=w226) -> ("k domain resampled"=w251:cluster{dbl[], "best nonlinear fit":dbl[]}[], "frequency domain info"=w243:T12)  [unwired: 5 in, 2 out]
              n50 = call "PSDLorentianFit_NODECIMATION_array_input.vi"("High frequency cutoff %"=w238, "dt [s]"=w254, "signal"=w225) -> ("k domain resampled"=w252:cluster{dbl[], "best nonlinear fit":dbl[]}[], "frequency domain info"=w242:T12)  [unwired: 5 in, 2 out]
              n51 = call-poly <vilib>:"Write Delimited Spreadsheet.vi"("file path (dialog if empty)"=w218, "format (%.3f)"="%.6e", "2D data"=w216) -> ()  [unwired: 11 in, 2 out]
              n52 = Reciprocal(x=w229) -> (1/x=w232:dbl)
              n53 = Unbundle By Name(w245) -> ("pi A^2/f0"=w236:dbl)
              n54 = Unbundle By Name(w244) -> ("pi A^2/f0"=w235:dbl)
              n55 = Unbundle By Name(w243) -> ("pi A^2/f0"=w234:dbl)
              n56 = Unbundle By Name(w242) -> ("pi A^2/f0"=w233:dbl)
              n57 = Index Array(array=w253) -> (element=w249:cluster{dbl[], "best nonlinear fit":dbl[]})  [unwired: 1 in]
              n58 = Index Array(array=w250) -> (element=w248:cluster{dbl[], "best nonlinear fit":dbl[]})  [unwired: 1 in]
              n59 = Index Array(array=w251) -> (element=w247:cluster{dbl[], "best nonlinear fit":dbl[]})  [unwired: 1 in]
              n60 = Index Array(array=w252) -> (element=w246:cluster{dbl[], "best nonlinear fit":dbl[]})  [unwired: 1 in]
            }
            n61 = Multiply(x=w182, y=w183) -> (x*y=w181:i32)
            n62 = Reciprocal(x=w156) -> (1/x=w161:dbl)
            n63 = Build Array(w169) -> (w168:dbl[][])
            n64 = Transpose 2D Array(2D array=w168) -> (transposed array=w167:dbl[][])
            n65 = Multiply(x=1000.0, y=w156) -> (x*y=w157:dbl)
            n66 = Format Value(string ("")="power=", format string="%dmW", value (0)=w157) -> (output string=w160:string)
            n67 = Concatenate Strings(w155, w160, w159) -> (w173:string)
            n68 = Build Path(base path=w172, name or relative path=w173) -> (appended path=w171:path)
            n69 = call-poly <vilib>:"Write Delimited Spreadsheet.vi"("file path (dialog if empty)"=w171, "format (%.3f)"="%.6e", "2D data"=w167) -> ()  [unwired: 11 in, 2 out]
            n70 = Build Array(w197, w198, w199, w201, w195) -> (w196:dbl[][])
            n71 = for {
              tunnel: w196 -> [w205] mode=indexing
              tunnel: [w206] -> w189 mode=indexing
              tunnel: w200 -> [w208]
              tunnel: [w207] -> w194 mode=indexing
              tunnel: [w204] -> w174 mode=indexing
              n72 = call <vilib>:"Median.vi"("X"=w205) -> ("median"=w206:dbl)  [unwired: 1 out]
              n73 = call <vilib>:"Std Deviation and Variance.vi"("X"=w205) -> ("variance"=w204:dbl)  [unwired: 1 in, 2 out]
              n74 = Bundle(w208, w205) -> (w207:cluster{dbl[], dbl[]})  [unwired: 1 in]
            }
            n75 = Index Array(array=w194) -> (element #1=w193:cluster{dbl[], dbl[]}, element #2=w192:cluster{dbl[], dbl[]}, element #3=w191:cluster{dbl[], dbl[]}, element #4=w190:cluster{dbl[], dbl[]})  [unwired: 4 in]
            n76 = Index Array(array=w189) -> (element #1=w184:dbl, element #2=w185:dbl, element #3=w186:dbl, element #4=w187:dbl, element #5=w188:dbl)  [unwired: 5 in]
          }
          n77 = Unbundle By Name(w106) -> ("height finder result"=w116:cluster{"Y":dbl[], "Y":dbl[]}[], "Z center positon"=w112:dbl, "Z signal Truncated data with redrawn polynomial"=w113:cluster{dbl[], "Best Polynomial Fit":dbl[]}[], "Instrument Calibr.XYZsignal baseline.Zsignal0"=w110:dbl, "X signal Truncated data with redrawn polynomial"=w109:cluster{dbl[], "Best Polynomial Fit":dbl[]}[])
          n78 = Unbundle By Name(w106) -> ("height finder result"=w148:cluster{"Y":dbl[], "Y":dbl[]}[], "Z signal Truncated data with redrawn polynomial"=w135:cluster{dbl[], "Best Polynomial Fit":dbl[]}[], "X signal Truncated data with redrawn polynomial"=w134:cluster{dbl[], "Best Polynomial Fit":dbl[]}[], "Y signal Truncated data with redrawn polynomial"=w133:cluster{dbl[], "Best Polynomial Fit":dbl[]}[])
          n79 = Index Array(array=w116) -> (element #1=w102:cluster{"Y":dbl[], "Y":dbl[]})  [unwired: 2 in, 1 out]
          n80 = Index Array(array=w109) -> (element=w108:cluster{dbl[], "Best Polynomial Fit":dbl[]})  [unwired: 1 in]
          n81 = Index Array(array=w113, index #2=3 ("index")) -> (element #1=w120:cluster{dbl[], "Best Polynomial Fit":dbl[]})  [unwired: 1 in, 1 out]
          n82 = Unbundle(w108) -> ("Best Polynomial Fit"=w107:dbl[])  [unwired: 1 out]
          n83 = Unbundle(w120) -> ("Best Polynomial Fit"=w119:dbl[])  [unwired: 1 out]
          n84 = Unbundle(w102) -> ("Y"=w115:dbl[])  [unwired: 1 out]
          n85 = Array Max & Min(array=w119) -> (min value=w118:dbl)  [unwired: 3 out]
          n86 = Array Max & Min "max x signal (to calculate max x force)"(array=w107) -> (max value=w103:dbl)  [unwired: 3 out]
          n87 = call "HeightFinder.Fit2.vi"("Vsum or Z signal"=w115, "Treat baseline parallel"=TRUE) -> ("bottom position"=w114:dbl)  [unwired: 1 in, 6 out]
          n88 = Index Array(array=w148) -> (element=w89:cluster{"Y":dbl[], "Y":dbl[]})  [unwired: 1 in]
          n89 = Index Array(array=w135, index=w126) -> (element=w85:cluster{dbl[], "Best Polynomial Fit":dbl[]})
          n90 = Index Array(array=w134, index=w126) -> (element=w83:cluster{dbl[], "Best Polynomial Fit":dbl[]})
          n91 = Index Array(array=w133, index=w126) -> (element=w82:cluster{dbl[], "Best Polynomial Fit":dbl[]})
          n92 = Subtract "max Delta z signal\n(to calculate max z force)"(x=w110, y=w118) -> (x-y=w104:dbl)
          n93 = Subtract(x=w114, y=w112) -> (x-y=→"distance between trap center and z DoG center":dbl)
          n94 = Bundle(w104, w103) -> (w99:cluster{dbl, dbl})  [unwired: 1 in]
          n95 = Unbundle By Name(w106) -> ("z_signal vs trap height slope around eq position, 1/nm"=w130:dbl, "x_signal vs trap height slope around eq position, 1/nm"=w131:dbl, "y_signal vs trap height slope around eq position, 1/nm"=w132:dbl)
          n96 = Index Array(array=w61) -> (element #1=→"ellipticity fitting":cluster{dbl[], "best nonlinear fit":dbl[]}[], element #2=→"ellipticity fitting 2":cluster{dbl[], "best nonlinear fit":dbl[]}[], element #3=→"ellipticity fitting 3":cluster{dbl[], "best nonlinear fit":dbl[]}[], element #4=→"ellipticity fitting 4":cluster{dbl[], "best nonlinear fit":dbl[]}[])  [unwired: 8 in]
          n97 = local read "result"() -> (w90:T2)
          n98 = Bundle(w62, w142) -> (w76:cluster{dbl[], dbl[]})  [unwired: 1 in]
          n99 = Bundle(w62, w141) -> (w75:cluster{dbl[], dbl[]})  [unwired: 1 in]
          n100 = Bundle(w62, w140) -> (w74:cluster{dbl[], dbl[]})  [unwired: 1 in]
          n101 = Bundle(w62, w63) -> (w73:cluster{dbl[], dbl[]})  [unwired: 1 in]
          n102 = Build Array(w85) -> (w86:cluster{dbl[], "Best Polynomial Fit":dbl[]}[])
          n103 = Build Array(w83) -> (w84:cluster{dbl[], "Best Polynomial Fit":dbl[]}[])
          n104 = Build Array(w82) -> (w81:cluster{dbl[], "Best Polynomial Fit":dbl[]}[])
          n105 = Reshape Array(w61, w136) -> (w68:cluster{dbl[], "best nonlinear fit":dbl[]}[])
          n106 = Reshape Array(w139, w136) -> (w67:cluster{dbl[], "best nonlinear fit":dbl[]}[])
          n107 = Reshape Array(w138, w136) -> (w66:cluster{dbl[], "best nonlinear fit":dbl[]}[])
          n108 = Reshape Array(w137, w136) -> (w65:cluster{dbl[], "best nonlinear fit":dbl[]}[])
          n109 = Build Array(w76) -> (w72:cluster{dbl[], dbl[]}[])
          n110 = Build Array(w75) -> (w71:cluster{dbl[], dbl[]}[])
          n111 = Build Array(w74) -> (w70:cluster{dbl[], dbl[]}[])
          n112 = Build Array(w73) -> (w69:cluster{dbl[], dbl[]}[])
          n113 = call-poly <vilib>:"Mean.vi"("X"=w124) -> ("mean"=w122:dbl)  [unwired: 1 out]
          n114 = Bundle(w129, w124) -> (w87:cluster{dbl[], dbl[]})  [unwired: 1 in]
          n115 = Build Array(w87) -> (w88:cluster{dbl[], dbl[]}[])
          n116 = Bundle(cluster=w90, "max ellipticity vs power"=w88, "z DoG"=w86, "x DoG"=w84, "y DoG"=w81, "ellipticity vs angle"=w80, "z variance vs angle"=w79, "x variance vs angle"=w78, "y variance vs angle"=w77, "var ellipticity vs power"=w72, "var z signal vs power"=w71, "var x signal vs power"=w70, "var y signal vs power"=w69, "ellipticity fitting"=w68, "z signal fitting"=w67, "x signal fitting"=w66, "y signal fitting"=w65) -> (w91:T2)
          n117 = local write "result"(w91) -> ()
          n118 = Multiply(x=w122, y=2.0 ("x")) -> (x*y=w123:dbl)
          n119 = Build Array(w123, w130, w131, w132) -> (w56:dbl[])
          n120 = Absolute Value(x=w56) -> (abs(x)=w55:dbl[])
          n121 = Bundle(w51, w89, w87, w85, w83, w82, w55, w80, w79, w78, w77, w99, w76, w75, w74, w73, w68, w67, w66, w65, w54) -> (w98:T13)  [unwired: 1 in]
          n122 = Build Array (concatenate)(w96, w98) -> (w97:T4)
          "data" <- w97
        }
        n123 = property class="LstBox (strict)"(reference=w44, error in=w42, "Item Names"=w36) -> (reference out=w47:refnum<vi>, error out=w46:errorcluster, "Item Symbols"=w45:i32[])
        n124 = for {
          tunnel: [0] -> w48 mode=indexing
          tunnel: w45 -> [_] mode=indexing
        }
        n125 = property class="LstBox (strict)"(reference=w47, error in=w46, "Item Symbols"=w48) -> (error out=w40:errorcluster)  [unwired: 1 out]
        n126 = local write "pb1"(w39) -> ()
      }
      event "cylinder list": Value Change {
        n127 = event-data() -> ("Type"=w260:T11)  [unwired: 1 in]
        n128 = stacked-sequence {
          seq-local: [w296 _ _] -> [_ w393 _]
          tunnel: w262 -> [_ _ w481]
          tunnel: [_ _ w480] -> w261
          frame #0 {
            (unwired) cluster{"order":i32, "coefficient":dbl}[] [{"order"=0, "coefficient"=0.0}] ("Coefficient Constraint")
            # "column name:\n\n0: Cylinder No.\n1: Good? (=1)\n2: K_theta\n3: S_theta\n4: K_e\n5: K_z\n6: S_z\n7: K_zsig\n8: K_x\n9: S_x\n10: K_xsig\n11: K_y\n12: S_y\n13: K_ysig\n14: Max z signal\n15: Max x signal"
            n129 = local read "data"() -> (w295:T4)
            n130 = for {
              tunnel: w295 -> [w329]
              tunnel: "cylinder list" -> [w328] mode=indexing
              tunnel: [w326] -> w293 mode=indexing
              tunnel: [w300] -> w291 mode=indexing
              tunnel: [w321] -> w292 mode=indexing
              tunnel: [w320] -> w290 mode=indexing
              tunnel: [w311] -> w289 mode=indexing
              tunnel: [w310] -> w288 mode=indexing
              tunnel: [w309] -> w280 mode=indexing
              tunnel: [w308] -> w279 mode=indexing
              tunnel: [w307] -> w278 mode=indexing
              tunnel: [w306] -> w277 mode=indexing
              tunnel: [w305] -> w283 mode=indexing
              tunnel: [w303] -> w282 mode=indexing
              tunnel: [w302] -> w281 mode=indexing
              tunnel: [w301] -> w272 mode=indexing
              n131 = Index Array(array=w329, index=w328) -> (element=w327:T14)
              n132 = Unbundle(w327) -> (w326:i32, w320:cluster{"Y":dbl[], "Y":dbl[]}, w309:cluster{dbl[], dbl[]}, w308:cluster{dbl[], "Best Polynomial Fit":dbl[]}, w307:cluster{dbl[], "Best Polynomial Fit":dbl[]}, w306:cluster{dbl[], "Best Polynomial Fit":dbl[]}, w305:dbl[], w315:cluster{dbl[], dbl[]}[], w314:cluster{dbl[], dbl[]}[], w313:cluster{dbl[], dbl[]}[], w312:cluster{dbl[], dbl[]}[], w304:cluster{dbl, dbl}, w325:cluster{dbl[], dbl[]}, w324:cluster{dbl[], dbl[]}, w323:cluster{dbl[], dbl[]}, w322:cluster{dbl[], dbl[]}, w319:cluster{dbl[], "best nonlinear fit":dbl[]}[], w318:cluster{dbl[], "best nonlinear fit":dbl[]}[], w317:cluster{dbl[], "best nonlinear fit":dbl[]}[], w316:cluster{dbl[], "best nonlinear fit":dbl[]}[], "var of linear fittings"=w299:dbl[][])
              n133 = Build Array(w315, w314, w313, w312) -> (w311:cluster{dbl[], dbl[]}[][])
              n134 = Build Array(w325, w324, w323, w322) -> (w301:cluster{dbl[], dbl[]}[])
              n135 = Build Array(w319, w318, w317, w316) -> (w310:cluster{dbl[], "best nonlinear fit":dbl[]}[][])
              n136 = Transpose 2D Array(2D array=w299) -> (transposed array=w298:dbl[][])
              n137 = Unbundle(w304) -> (w303:dbl, w302:dbl)
              n138 = for "different signals" {
                tunnel: w301 -> [w338] mode=indexing
                tunnel: [w336] -> w300 mode=indexing
                tunnel: [w337] -> w321 mode=indexing
                tunnel: w298 -> [w335] mode=indexing
                n139 = Reciprocal(x=w335) -> (1/x=w330:dbl[])
                n140 = Unbundle(w338) -> (w331:dbl[], w332:dbl[])
                n141 = call <vilib>:"General Polynomial Fit.vi"("Y"=w332, "polynomial order"=1, "X"=w331, "Weight"=w330) -> ("Polynomial Coefficients"=w333:dbl[])  [unwired: 8 in, 3 out]
                n142 = Index Array(array=w333) -> (element #1=w337:dbl, element #2=w336:dbl)  [unwired: 2 in]
              }
            }
            "only use slopes" <- w291
            "intercepts that will be ignored" <- w292
            "Height finder data" <- w290
            n143 = Transpose 2D Array(2D array=w272) -> (transposed array=w271:cluster{dbl[], dbl[]}[][])
            n144 = Index Array(array=w289) -> (element=w286:cluster{dbl[], dbl[]}[][])  [unwired: 3 in]
            n145 = Index Array(array=w288) -> (element=w287:cluster{dbl[], "best nonlinear fit":dbl[]}[][])  [unwired: 3 in]
            n146 = Index Array(array=w286) -> (element #1=w276:cluster{dbl[], dbl[]}[], element #2=w273:cluster{dbl[], dbl[]}[], element #3=w274:cluster{dbl[], dbl[]}[], element #4=w275:cluster{dbl[], dbl[]}[])  [unwired: 8 in]
            n147 = Index Array(array=w271) -> (element #1=w270:cluster{dbl[], dbl[]}[], element #2=w269:cluster{dbl[], dbl[]}[], element #3=w267:cluster{dbl[], dbl[]}[], element #4=w268:cluster{dbl[], dbl[]}[])  [unwired: 8 in]
            n148 = Index Array(array=w287) -> (element #1=w263:cluster{dbl[], "best nonlinear fit":dbl[]}[], element #2=w264:cluster{dbl[], "best nonlinear fit":dbl[]}[], element #3=w265:cluster{dbl[], "best nonlinear fit":dbl[]}[], element #4=w266:cluster{dbl[], "best nonlinear fit":dbl[]}[])  [unwired: 8 in]
            n149 = local read "result"() -> (w284:T2)
            n150 = Bundle(cluster=w284, "max ellipticity vs power"=w280, "z DoG"=w279, "x DoG"=w278, "y DoG"=w277, "ellipticity vs angle"=w276, "z variance vs angle"=w273, "x variance vs angle"=w274, "y variance vs angle"=w275, "var ellipticity vs power"=w270, "var z signal vs power"=w269, "var x signal vs power"=w267, "var y signal vs power"=w268, "ellipticity fitting"=w263, "z signal fitting"=w264, "x signal fitting"=w265, "y signal fitting"=w266) -> (→"result":T2)
            n151 = for {
              tunnel: w291 -> [w348] mode=indexing
              tunnel: w283 -> [w342] mode=indexing
              tunnel: "kT_pNnm" -> [w347]
              tunnel: w282 -> [w344] mode=indexing
              tunnel: w293 -> [w346] mode=indexing
              tunnel: [w343] -> w296 mode=indexing
              tunnel: w281 -> [w340] mode=indexing
              tunnel: [w339] -> _ mode=indexing
              i -> [w339]
              n152 = Square(x=w342) -> (x^2=w351:dbl[])
              n153 = Divide(x=w348, y=w351) -> (x/y=w352:dbl[])
              n154 = Divide "k_theta"(x=w347, y=w352) -> (x/y=w350:dbl[])
              n155 = Divide "K_e"(x=w350, y=w342) -> (x/y=w349:dbl[])
              n156 = Interleave 1D Arrays(w350, w342, w349) -> (w345:dbl[])
              n157 = Build Array (concatenate)(w346, nan ("element"), w345, w344, w340) -> (w343:dbl[])
            }
            "Array" <- w296
          }
          frame #1 {
            # "column name:\n\n0: Cylinder No.\n1: Good? (=1)\n2: K_theta\n3: S_theta\n4: K_e\n5: K_z\n6: S_z\n7: K_zsig\n8: K_x\n9: S_x\n10: K_xsig\n11: K_y\n12: S_y\n13: K_ysig\n14: Max z signal\n15: Max x signal"
            n158 = Transpose 2D Array(2D array=w393) -> (transposed array=w427:dbl[][])
            "final result" <- w427
            n159 = Array Size(array=w393) -> (size(s)=w394:i32[])
            n160 = Index Array(array=w393, index (col) #1=0 ("disabled index (col)"), index (col) #2=4 ("disabled index (col)"), index (col) #3=7 ("index (col)"), index (col) #4=3 ("index (col)"), index (col) #5=6 ("index (col)"), index (col) #6=2 ("index (col)"), index (col) #7=5 ("index (col)"), index (col) #8=9 ("index (col)"), index (col) #9=8 ("index (col)"), index (col) #10=10 ("index (col)")) -> (element #1=w384:dbl[], element #2=w410:dbl[], element #3=w389:dbl[], element #4=w417:dbl[], element #5=w418:dbl[], element #6=w454:dbl[], element #7=w451:dbl[], element #8=w378:dbl[], element #9=w379:dbl[], element #10=w380:dbl[])  [unwired: 10 in]
            n161 = Index Array(array=w394, index=1) -> (element=w396:i32)
            n162 = Decrement(x=w396) -> (x-1=w391:i32)
            n163 = Decrement(x=w391) -> (x-1=w392:i32)
            n164 = for {
              N -> [w479]
              tunnel: w427 -> [w478] mode=indexing
              tunnel: [w479] -> w397
              tunnel: [w477] -> w354 mode=indexing
              tunnel: [w476] -> w353 mode=indexing
              n165 = call <vilib>:"Std Deviation and Variance.vi"("X"=w478) -> ("mean"=w477:dbl, "standard deviation"=w476:dbl)  [unwired: 1 in, 1 out]
            }
            "mean" <- w354
            "sd" <- w353
            n166 = Divide(x=w454, y=2 ("index")) -> (x/y=w456:dbl[])
            n167 = Index Array(array=w393, index (col) #1=w392, index (col) #2=w391) -> (element #1=w390:dbl[], element #2=w388:dbl[])  [unwired: 2 in]
            n168 = Multiply(x=w389, y=w390) -> (x*y=w458:dbl[])
            n169 = Multiply(x=w389, y=w388) -> (x*y=w371:dbl[])
            n170 = Bundle(w384, w410) -> (→"Torque sensitivity":cluster{dbl[], dbl[]})  [unwired: 1 in]
            n171 = Bundle(w384, w389) -> (→"z force sensitivity":cluster{dbl[], dbl[]})  [unwired: 1 in]
            n172 = Bundle(w384, w417) -> (→"Angular sensitivity":cluster{dbl[], dbl[]})  [unwired: 1 in]
            n173 = Bundle(w384, w418) -> (→"z sensitivity":cluster{dbl[], dbl[]})  [unwired: 1 in]
            n174 = Bundle(w384, w454) -> (→"Angular stiffness":cluster{dbl[], dbl[]})  [unwired: 1 in]
            n175 = Bundle(w384, w451) -> (→"z stiffness":cluster{dbl[], dbl[]})  [unwired: 1 in]
            n176 = Bundle(w384, w378) -> (→"x sensitivity":cluster{dbl[], dbl[]})  [unwired: 1 in]
            n177 = Bundle(w384, w379) -> (→"x stiffness":cluster{dbl[], dbl[]})  [unwired: 1 in]
            n178 = Bundle(w384, w380) -> (→"x force sensitivity":cluster{dbl[], dbl[]})  [unwired: 1 in]
            n179 = Bundle(w384, w456) -> (→"Maximum torque":cluster{dbl[], dbl[]})  [unwired: 1 in]
            n180 = Bundle(w384, w458) -> (→"Maximum z force":cluster{dbl[], dbl[]})  [unwired: 1 in]
            n181 = Bundle(w384, w371) -> (→"Maximum x force":cluster{dbl[], dbl[]})  [unwired: 1 in]
            n182 = Square Root(x=w397) -> (sqrt(x)=w372:dbl)
            n183 = call <vilib>:"Std Deviation and Variance.vi"("X"=w458) -> ("mean"=w461:dbl, "standard deviation"=w460:dbl)  [unwired: 1 in, 1 out]
            "max z force, pN/W" <- w461
            "SD of max z force, pN/W" <- w460
            n184 = call <vilib>:"Std Deviation and Variance.vi"("X"=w371) -> ("mean"=w375:dbl, "standard deviation"=w374:dbl)  [unwired: 1 in, 1 out]
            "max x force, pN/W" <- w375
            "SD of max x force, pN/W" <- w374
            n185 = Divide(x=w353, y=w372) -> (x/y=w398:dbl[])
            n186 = Divide(x=w353, y=w354) -> (x/y=w469:dbl[])
            n187 = Divide(x=w460, y=w372) -> (x/y=→"SEM of max z force, pN/W":dbl)
            n188 = Divide(x=w460, y=w461) -> (x/y=→"CV of max z force":dbl)
            n189 = Divide(x=w374, y=w372) -> (x/y=→"SEM of max x force, pN/W":dbl)
            n190 = Divide(x=w374, y=w375) -> (x/y=→"CV of max x force":dbl)
            n191 = Index Array(array=w354, index #1=3 ("index"), index #2=2 ("index"), index #3=6 ("index"), index #4=5 ("index"), index #5=4 ("index"), index #6=7 ("index"), index #7=8 ("index (col)"), index #8=9 ("index (col)")) -> (element #1=→"mean angular sensitivity, 1/rad":dbl, element #2=→"mean angular stiffness, pNnm/rad/W":dbl, element #3=→"mean z sensitivity, 1/nm":dbl, element #4=→"mean z stiffness, pN/nm/W":dbl, element #5=→"mean torque sensitivity, pNnm/W":dbl, element #6=→"mean force sensitivity, pN/W":dbl, element #7=→"mean x stiffness, pN/nm/W":dbl, element #8=→"mean z sensitivity, 1/nm 2":dbl)
            n192 = Index Array(array=w398, index #1=3 ("index"), index #2=2 ("index"), index #3=6 ("index"), index #4=5 ("index"), index #5=4 ("index"), index #6=7 ("index"), index #7=8 ("index (col)"), index #8=9 ("index (col)")) -> (element #1=→"SEM of angular sensitivity, 1/rad":dbl, element #2=→"SEM of angular stifness, pNnm/rad/W":dbl, element #3=→"SEM of z sensitivity, 1/nm":dbl, element #4=→"SEM of z stiffness, pN/nm/W":dbl, element #5=→"SEM of torque sensitivity, pNnm/W":dbl, element #6=→"SEM of force sensitivity, pN/W":dbl, element #7=→"SEM of x stiffness, pN/nm/W":dbl, element #8=→"SEM of z sensitivity, 1/nm 2":dbl)
            n193 = Index Array(array=w353, index #1=3 ("index"), index #2=2 ("index"), index #3=6 ("index"), index #4=5 ("index"), index #5=4 ("index"), index #6=7 ("index"), index #7=8 ("index (col)"), index #8=9 ("index (col)")) -> (element #1=→"SD of angular sensitivity, 1/rad":dbl, element #2=→"SD of angular stifness, pNnm/rad/W":dbl, element #3=→"SD of z sensitivity, 1/nm":dbl, element #4=→"SD of z stiffness, pN/nm/W":dbl, element #5=→"SD of torque sensitivity, pNnm/W":dbl, element #6=→"SD of force sensitivity, pN/W":dbl, element #7=→"SD of x stiffness, pN/nm/W":dbl, element #8=→"SD of z sensitivity, 1/nm 2":dbl)
            n194 = Index Array(array=w469, index #1=3 ("index"), index #2=2 ("index"), index #3=6 ("index"), index #4=5 ("index"), index #5=4 ("index"), index #6=7 ("index"), index #7=8 ("index (col)"), index #8=9 ("index (col)")) -> (element #1=→"CV of angular sensitivity":dbl, element #2=→"CV of angular stifness":dbl, element #3=→"CV of z sensitivity":dbl, element #4=→"CV of z stiffness":dbl, element #5=→"CV of torque sensitivity":dbl, element #6=→"CV of force sensitivity":dbl, element #7=→"CV of x stiffness":dbl, element #8=→"CV of z sensitivity 2":dbl)
          }
          frame #2 {
            w492 = "[Comment from " ("search string")
            n195 = local read "mean angular stiffness, pNnm/rad/W"() -> (w518:dbl)
            n196 = local read "mean z stiffness, pN/nm/W"() -> (w519:dbl)
            n197 = local read "mean z sensitivity, 1/nm"() -> (w517:dbl)
            n198 = local read "mean angular sensitivity, 1/rad"() -> (w515:dbl)
            n199 = local read "original calibration file"() -> (w486:string)
            n200 = local read "mean"() -> (w512:dbl[])
            n201 = Index Array(array=w512, index #1=8, index #2=9, index #3=11, index #4=12) -> (element #1=w507:dbl, element #2=w506:dbl, element #3=w505:dbl, element #4=w504:dbl)
            n202 = Build Array(w507, w506, w505, w504) -> (w503:dbl[])
            n203 = Divide(x=w515, y=2.0) -> (x/y=w514:dbl)
            n204 = Build Array("Kz, pN/nm/W=", "Kang, pNnm/rad/W=", "Sz, 1/nm=", "Max ellipticity, 1=", "Kx, pN/nm/W=", "Sx, 1/nm=", "Ky, pN/nm/W=", "Sy, 1/nm=") -> (w520:string[])
            n205 = Build Array (concatenate)(w519, w518, w517, w514, w503) -> (w516:dbl[])
            n206 = local read "Name"() -> (w484:string)
            n207 = local read "Comment"() -> (w483:string)
            n208 = for {
              tunnel: w520 -> [w552] mode=indexing
              tunnel: w516 -> [w549] mode=indexing
              shift-right: [w545] -> w496
              shift-left: w486 -> [w555]
              n209 = Search/Split String(string=w555, search string/char (-)=w552) -> (substring before match=w553:string, match + rest of string=w551:string)  [unwired: 1 in, 1 out]
              n210 = Search and Replace String(input string=w551, search string=w552) -> (result string=w550:string)  [unwired: 6 in, 3 out]
              n211 = Scan Value(string=w550, format string="%f", default (0 dbl)=w549) -> (output string=w546:string)  [unwired: 1 out]
              n212 = Format Value(format string="%.6f", value (0)=w549) -> (output string=w547:string)  [unwired: 1 in]
              n213 = Concatenate Strings(w553, w552, w547, w546) -> (w545:string)
            }
            n214 = local read "Updated calibration file location"() -> (w485:path)
            n215 = Get Date/Time String() -> (date string=w491:string, time string=w489:string)  [unwired: 3 in]
            n216 = Search and Replace String(input string=w496, search string=w492, replace string=w492) -> (result string=w497:string, number of replacements=w493:i32, offset past replacement=w498:i32)  [unwired: 5 in, 1 out]
            n217 = case shown="..0" w493 {
              tunnel: w498 -> [_ w533]
              tunnel: w497 -> [w526 w532]
              tunnel: [w527 w530] -> w487
              tunnel: w492 -> [w528 _]
              frame ..0 {
                n218 = call <vilib>:"Trim Whitespace.vi"("string"=w526) -> ("trimmed string"=w525:string)  [unwired: 1 in]
                n219 = Concatenate Strings(w525, "\r\n", w528) -> (w527:string)
              }
              frame 1.. {
                n220 = String Subset(string=w532, offset (0)=0, length (rest)=w533) -> (substring=w530:string)
              }
            }
            n221 = Concatenate Strings(w487, w484, "] " ("string"), w483, "\r\n", w491, " ", w489) -> (w495:string)
            n222 = case shown="No Error" w481 {
              selector: w481 -> [w541 w543]
              tunnel: w495 -> [w535 _]
              tunnel: w485 -> [w542 _]
              tunnel: [w535 "Error! file doesn't exist"] -> w482
              tunnel: [w534 w543] -> w480
              frame No Error {
                n223 = Write to Text File(file (use dialog)=w542, text=w535, error in=w541) -> (refnum out=w537:refnum<file>, error out=w539:errorcluster)  [unwired: 1 in, 1 out]
                n224 = Deny Access(4:w539, 6:T10."deny write-only" ("deny mode (0:deny read/write)"), 7:w537) -> (0:w538:errorcluster, 3:w536:refnum<file>)
                n225 = Close File(refnum=w536, error in=w538) -> (error out=w534:errorcluster)  [unwired: 1 out]
              }
              frame Error {
              }
            }
            "Updated calibration file" <- w482
          }
        }
      }
      event "stop": Value Change; Panel Close {
        n226 = event-data() -> ("Type"=w556:T11)  [unwired: 1 in]
      }
    }
    "error out" <- w30
  }
